vi "Configure Harmonics Measure Step.vi"(8 "error in (no error)":errorcluster, 9 "SA Pin":string, 10 "Harmonic Order":i8, 11 "Harmonics in":refnum<class "Harmonics.lvclass">) -> (0 "error out":errorcluster, 2 "Result Name":string, 3 "Harmonics out":refnum<class "Harmonics.lvclass">)   [LabVIEW 2018, in "Harmonics.lvlib" / "Harmonics.lvclass"]
uses:
  Harmonics.lvclass
  C:/Sequence Automation/Plugins/Measurement Interface.lvlibp/Measurement Interface.lvclass
  Plugins/Measurement Interface.lvlibp/Private Methods/Engine Reference/Read Engine Reference.vi
  Plugins/Measurement Interface.lvlibp/Private Methods/Measurement Name/Read Measurement Name.vi
  Plugins/TestStand API Tools (TSAT).lvlibp/Step Actions/TSAT Step Actions.lvlib
  Plugins/Measurement Interface.lvlibp/Measurement Interface.lvclass
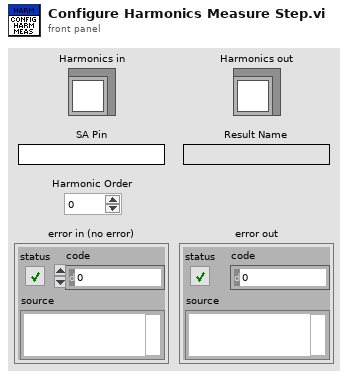
[diagram p1: front panel]
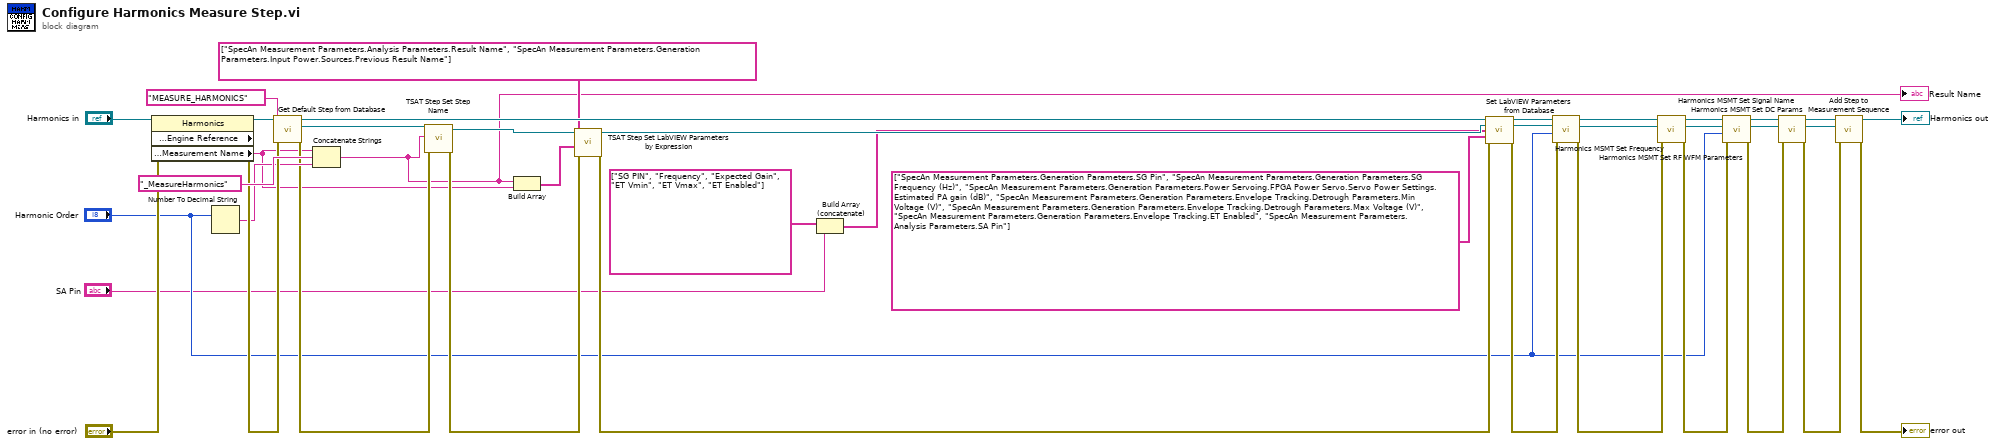
[diagram p0: block diagram]
diagram:
  n1 = property class="Harmonics" props=["Protected Methods:Engine Reference", "Public Methods:Measurement Name"](reference="Harmonics in", error in="error in (no error)") -> (reference out=w34:refnum<class "Harmonics.lvclass">, error out=w35:errorcluster, "Public Methods:Measurement Name"=w6:string)  [unwired: 1 out]
  n2 = Number To Decimal String(number="Harmonic Order") -> (decimal integer string=w32:string)  [unwired: 1 in]
  n3 = call "Get Default Step from Database.vi"("error in (no error)"=w35, "Default Step"="MEASURE_HARMONICS", "Measurement Interface in"=w34) -> ("error out"=w30:errorcluster, "Cloned Step"=w31:refnum<k7>, "Measurement Interface out"=w29:refnum<class "Harmonics.lvclass">)  [unwired: 6 in]
  n4 = Concatenate Strings(w6, "_MeasureHarmonics" ("string"), w32) -> (w5:string)
  "Result Name" <- w5
  n5 = call "TSAT Step Set Step Name.vi"("Error In"=w30, "Name"=w5, "Step In"=w31) -> ("Error Out"=w28:errorcluster, "Step Out"=w23:refnum<k7>)  [unwired: 7 in]
  n6 = Build Array(w5, w6) -> (w20:string[])
  n7 = call "TSAT Step Set LabVIEW Parameters by Expression.vi"("Error In"=w28, "Value Expressions"=w20, "Parameters to Set"=string[] ["SpecAn Measurement Parameters.Analysis Parameters.Result Name", "SpecAn Measurement Parameters.Generation Parameters.Input Power.Sources.Previous Result Name"], "Step In"=w23) -> ("Error Out"=w24:errorcluster, "Step Out"=w22:refnum<k7>)  [unwired: 6 in]
  n8 = Build Array (concatenate)(string[] ["SG PIN", "Frequency", "Expected Gain", "ET Vmin", "ET Vmax", "ET Enabled"] ("Database Keys"), "SA Pin") -> (w2:string[])
  n9 = call "Set LabVIEW Parameters from Database.vi"("Measurement Interface in"=w29, "Step In"=w22, "Dictionary Keys"=w2, "LabVIEW Parameter Mapping"=string[] ["SpecAn Measurement Parameters.Generation Parameters.SG Pin", "SpecAn Measurement Parameters.Generation Parameters.SG Frequency (Hz)", "SpecAn Measurement Parameters.Generation Parameters.Power Servoing.FPGA Power Servo.Servo Power Settings.Estimated PA gain (dB)", "SpecAn Measurement Parameters.Generation Parameters.Envelope Tracking.Detrough Parameters.Min Voltage (V)", "SpecAn Measurement Parameters.Generation Parameters.Envelope Tracking.Detrough Parameters.Max Voltage (V)", "SpecAn Measurement Parameters.Generation Parameters.Envelope Tracking.ET Enabled", "SpecAn Measurement Parameters.Analysis Parameters.SA Pin"] ("Database Keys"), "error in (no error)"=w24) -> ("Measurement Interface out"=w17:refnum<class "Harmonics.lvclass">, "Step Out"=w16:refnum<k7>, "error out"=w27:errorcluster)  [unwired: 8 in]
  n10 = call "Harmonics MSMT Set Frequency.vi"("error in (no error)"=w27, "Harmonic Order"="Harmonic Order", "Step In"=w16, "Harmonics in"=w17) -> ("error out"=w18:errorcluster, "Step Out"=w3:refnum<k7>, "Harmonics out"=w4:refnum<class "Harmonics.lvclass">)  [unwired: 5 in]
  n11 = call "Harmonics MSMT Set RF WFM Parameters.vi"("error in (no error)"=w18, "Step In"=w3, "Harmonics in"=w4) -> ("error out"=w19:errorcluster, "Step Out"=w13:refnum<k7>, "Harmonics MSMT out"=w14:refnum<class "Harmonics.lvclass">)  [unwired: 6 in]
  n12 = call "Harmonics MSMT Set Signal Name.vi"("error in (no error)"=w19, "Harmonic Order"="Harmonic Order", "Step In"=w13, "Harmonics in"=w14) -> ("error out"=w15:errorcluster, "Step Out"=w8:refnum<k7>, "Harmonics out"=w10:refnum<class "Harmonics.lvclass">)  [unwired: 5 in]
  n13 = call "Harmonics MSMT Set DC Params.vi"("error in (no error)"=w15, "Step In"=w8, "Harmonics in"=w10) -> ("error out"=w11:errorcluster, "Step Out"=w7:refnum<k7>, "Harmonics out"=w9:refnum<class "Harmonics.lvclass">)  [unwired: 6 in]
  n14 = call "Add Step to Measurement Sequence.vi"("error in (no error)"=w11, "Step to Add"=w7, "Measurement Interface in"=w9) -> ("error out"=→"error out":errorcluster, "Measurement Interface out"=→"Harmonics out":refnum<class "Harmonics.lvclass">)  [unwired: 7 in]
